vi "Rinocloud_HTTP_children_to_tree.vi"(8 "error in (no error)":errorcluster, 9 "Pagination variables":cluster{"limit":dbl, "offset":dbl}={"limit"=15.0, "offset"=0.0}, 10 "id":string, 11 "Tree Ref in":refnum<vi>) -> (0 "error out":errorcluster, 2 "Status":T1={"headers"="", "body"="", "ID"="", "Saved"=TRUE}, 3 "Tree Ref out":refnum<vi>)   [LabVIEW 2013, in "Rinocloud Library.lvlib"]
uses:
  Rinocloud Library.lvlib
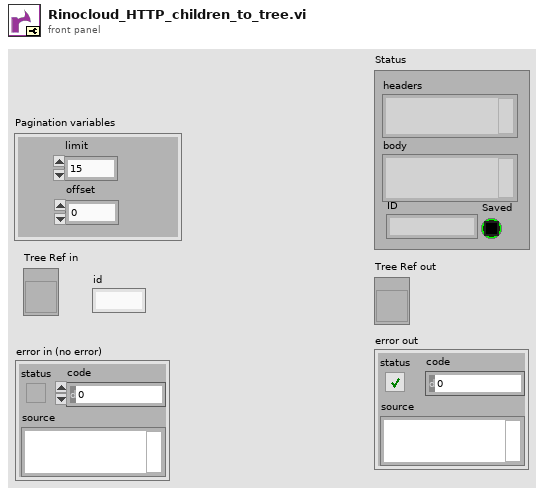
[diagram p1: front panel]
types:
  T1 = cluster{"headers":string, "body":string, "ID":string, "Saved":bool}
  T2 = cluster{"id":string, "name":string, "created_on":string, "updated_on":string, "tags":string, "notes":string, "record type":string, "metadata (JSON)":string, "project_name":string, "owner":string}[]
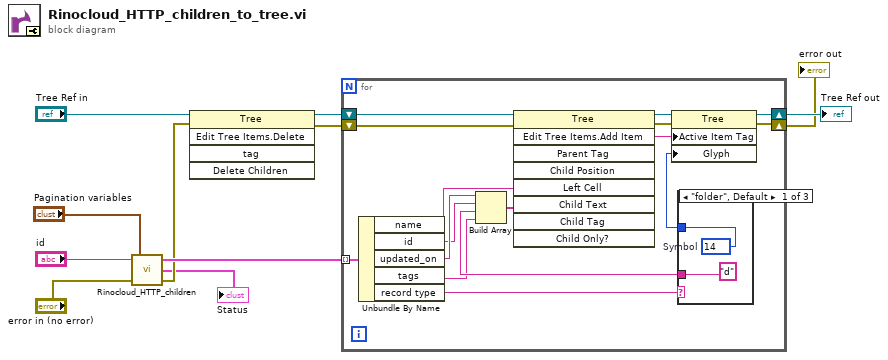
[diagram p0: block diagram]
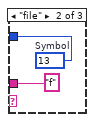
[diagram p2: hidden frame]
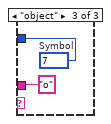
[diagram p3: hidden frame]
diagram:
  n1 = call "Rinocloud_HTTP_children.vi"("error in (no error)"="error in (no error)", "Pagination variables"="Pagination variables", "id"="id") -> ("error out"=w6:errorcluster, "Status"=→"Status":T1, "metadata array"=w8:T2)
  n2 = invoke class="Tree" method="Edit Tree Items.Delete"(reference="Tree Ref in", error in=w6) -> (reference out=w9:refnum<vi>, error out=w5:errorcluster)  [unwired: 3 in, 3 out]
  n3 = for {
    shift-right: [w24] -> w7
    shift-left: w9 -> [w26]
    tunnel: w8 -> [w27] mode=indexing
    shift-right: [w19] -> w3
    shift-left: w5 -> [w22]
    n4 = Unbundle By Name(w27) -> ("name"=w15:string, "id"=w14:string, "updated_on"=w16:string, "tags"=w12:string, "record type"=w18:string)
    n5 = case shown="\"folder\", Default" w18 {
      tunnel: [w29 w31 w32] -> w25
      tunnel: ["d" ("Parameter Name") "f" ("Parameter Name") "o" ("Parameter Name")] -> w13
      frame "folder", Default {
        w29 = 14  # Symbol
      }
      frame "file" {
        w31 = 13  # Symbol
      }
      frame "object" {
        w32 = 7  # Symbol
      }
    }
    n6 = Build Array(w16, w14, w13, w12) -> (w17:string[])
    n7 = invoke class="Tree" method="Edit Tree Items.Add Item"(reference=w26, error in=w22, "Left Cell"=w15, "Child Text"=w17) -> (reference out=w23:refnum<vi>, error out=w21:errorcluster, "Edit Tree Items:Add Item"=w20:string)  [unwired: 5 in, 6 out]
    n8 = property class="Tree"(reference=w23, error in=w21, "Active Item Tag"=w20, "Glyph"=w25) -> (reference out=w24:refnum<vi>, error out=w19:errorcluster)
  }
  "Tree Ref out" <- w7
  "error out" <- w3
